vi "ReadBGorCali (SubVI).vi"(7 "DataType":enum16{"BG", "Cali"}(ring), 8 "error in (no error)":errorcluster, 11 "file path in":path) -> (0 "error out":errorcluster, 2 "CtrlVCluster":T1, 3 "AvgDataCluster":T2)   [LabVIEW 2020]
panel:
  out "Waveform Graph":dbl[][](graph)
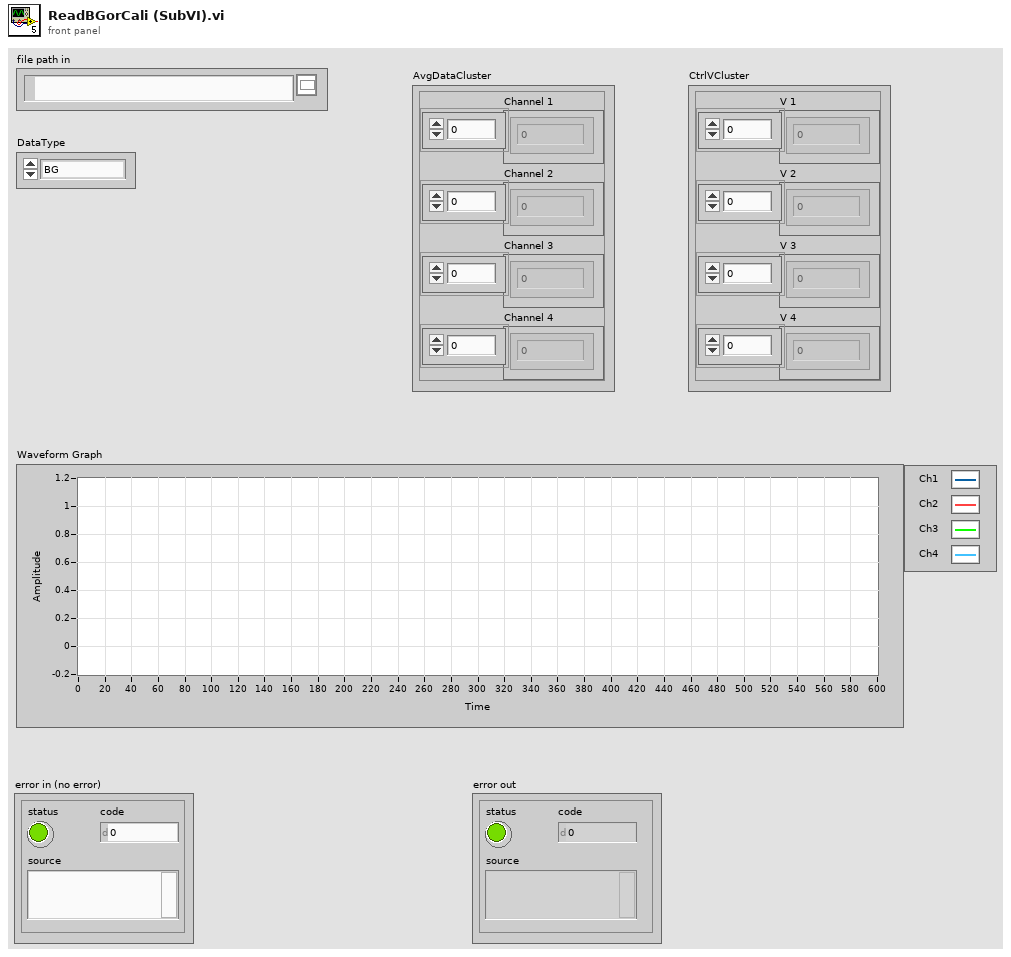
[diagram p1: front panel]
types:
  T1 = cluster{"V 1":dbl[], "V 2":dbl[], "V 3":dbl[], "V 4":dbl[]}
  T2 = cluster{"Channel 1":dbl[], "Channel 2":dbl[], "Channel 3":dbl[], "Channel 4":dbl[]}
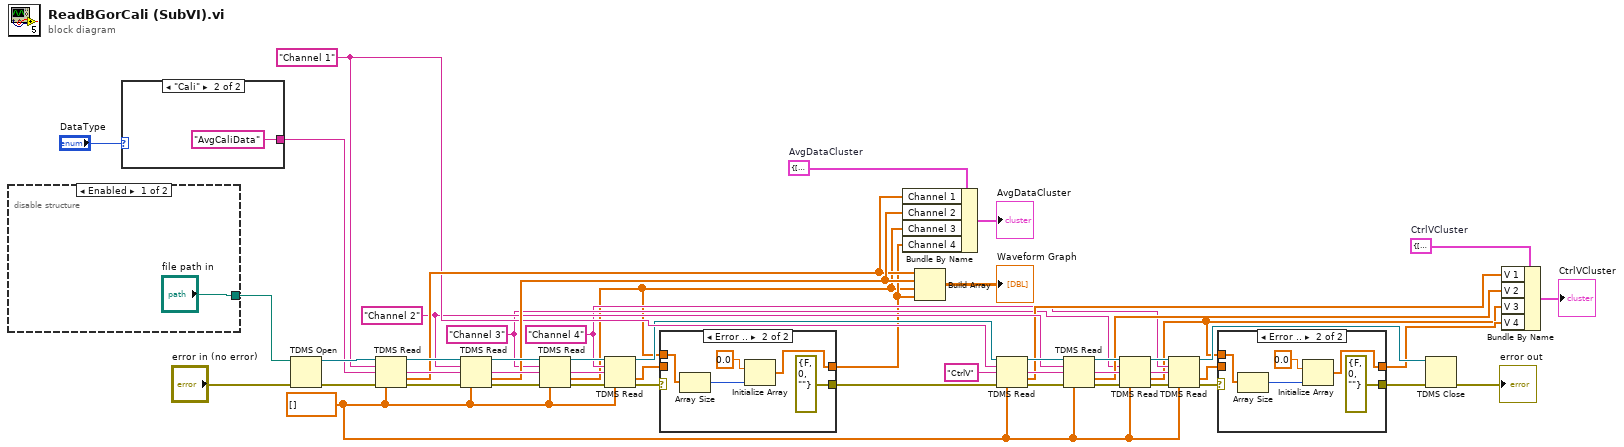
[diagram p0: block diagram]
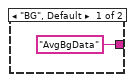
[diagram p4: hidden frame]
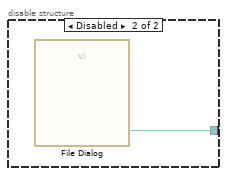
[diagram p5: hidden frame]
diagram:
  w13 = "Channel 4" ("group name in")
  w22 = T2 {"Channel 1"=[], "Channel 2"=[], "Channel 3"=[], "Channel 4"=[]}  # AvgDataCluster
  w24 = T1 {"V 1"=[], "V 2"=[], "V 3"=[], "V 4"=[]}  # CtrlVCluster
  w18 = "Channel 3" ("group name in")
  w30 = "Channel 2" ("group name in")
  w12 = dbl[] []
  w33 = "Channel 1" ("group name in")
  n1 = disable-structure shown="Enabled" {
    disable-tunnel: ["file path in" w54] -> w49
    frame Enabled {
    }
    frame Disabled {
      n2 = call "File Dialog"() -> ("selected path"=w54:path)  [unwired: 12 in, 3 out]
    }
  }
  n3 = case shown="\"Cali\"" "DataType" {
    tunnel: ["AvgBgData" "AvgCaliData"] -> w25
    frame "BG", Default {
    }
    frame "Cali" {
    }
  }
  n4 = TDMS Open(8:"error in (no error)", 11:w49) -> (0:w51:errorcluster, 3:w52:refnum<k34>)  [unwired: 5 in]
  n5 = TDMS Read(0:w52, 5:w33, 7:w25, 11:w51, 12:w12) -> (4:w48:refnum<k34>, 8:w46:string, 10:w39:dbl[], 15:w47:errorcluster)  [unwired: 3 in, 2 out]
  n6 = TDMS Read(0:w48, 5:w30, 7:w46, 11:w47, 12:w12) -> (4:w45:refnum<k34>, 8:w43:string, 10:w41:dbl[], 15:w44:errorcluster)  [unwired: 3 in, 2 out]
  n7 = TDMS Read(0:w45, 5:w18, 7:w43, 11:w44, 12:w12) -> (4:w21:refnum<k34>, 8:w19:string, 10:w2:dbl[], 15:w17:errorcluster)  [unwired: 3 in, 2 out]
  n8 = TDMS Read(0:w21, 5:w13, 7:w19, 11:w17, 12:w12) -> (4:w20:refnum<k34>, 10:w9:dbl[], 15:w10:errorcluster)  [unwired: 3 in, 3 out]
  n9 = case shown="Error .." w10 {
    selector: w10 -> [w57 _]
    tunnel: w9 -> [w58 _]
    tunnel: [w58 w59] -> w8
    tunnel: [w57 errorcluster {"status"=FALSE, "code"=0, "source"=""} ("error IO")] -> w7
    tunnel: w2 -> [_ w61]
    frame No Error {
    }
    frame Error {
      n10 = Array Size(array=w61) -> (size(s)=w60:i32)
      n11 = Initialize Array(0.0 ("element"), w60) -> (w59:dbl[])
    }
  }
  n12 = Bundle By Name(cluster=w22, "Channel 1"=w39, "Channel 2"=w41, "Channel 3"=w2, "Channel 4"=w8) -> (→"AvgDataCluster":T2)
  n13 = Build Array(w39, w41, w2, w8) -> (→"Waveform Graph":dbl[][])
  n14 = TDMS Read(0:w20, 5:w33, 7:"CtrlV" ("group name in"), 11:w7, 12:w12) -> (4:w38:refnum<k34>, 8:w32:string, 10:w29:dbl[], 15:w36:errorcluster)  [unwired: 3 in, 2 out]
  n15 = TDMS Read(0:w38, 5:w30, 7:w32, 11:w36, 12:w12) -> (4:w37:refnum<k34>, 8:w31:string, 10:w28:dbl[], 15:w35:errorcluster)  [unwired: 3 in, 2 out]
  n16 = TDMS Read(0:w37, 5:w18, 7:w31, 11:w35, 12:w12) -> (4:w16:refnum<k34>, 8:w14:string, 10:w1:dbl[], 15:w15:errorcluster)  [unwired: 3 in, 2 out]
  n17 = TDMS Read(0:w16, 5:w13, 7:w14, 11:w15, 12:w12) -> (4:w11:refnum<k34>, 10:w5:dbl[], 15:w6:errorcluster)  [unwired: 3 in, 3 out]
  n18 = case shown="Error .." w6 {
    selector: w6 -> [w64 _]
    tunnel: w5 -> [w65 _]
    tunnel: [w65 w66] -> w4
    tunnel: [w64 errorcluster {"status"=FALSE, "code"=0, "source"=""} ("error IO")] -> w3
    tunnel: w1 -> [_ w68]
    frame No Error {
    }
    frame Error {
      n19 = Array Size(array=w68) -> (size(s)=w67:i32)
      n20 = Initialize Array(0.0 ("element"), w67) -> (w66:dbl[])
    }
  }
  n21 = TDMS Close(8:w3, 11:w11) -> (0:→"error out":errorcluster)  [unwired: 1 out]
  n22 = Bundle By Name(cluster=w24, "V 1"=w29, "V 2"=w28, "V 3"=w1, "V 4"=w4) -> (→"CtrlVCluster":T1)
